vi "RollerTactic.vi"(7 "first call":bool, 8 "error in (no error)":errorcluster, 9 "Robot":refnum<class "Robot.lvclass">, 10 "Game in":refnum<class "Game.lvclass">, 11 "RollerTactic in":refnum<class "RollerTactic.lvclass">) -> (0 "error out":errorcluster, 2 "Robot out":refnum<class "Robot.lvclass">, 3 "RollerTactic out":refnum<class "RollerTactic.lvclass">)   [LabVIEW 2023, in "RollerTactic.lvclass"]
uses:
  RollerTactic.lvclass
  Robot_class/Robot.lvclass
  Game_class/Game.lvclass
  Robot_class/tactics.ctl
  Tactic_class/Tactic.lvclass/Tactic.ctl
  Game_class/Game.lvclass/Game.ctl
  Object_class/Object.lvclass/Object.ctl
  Skillbook_class/Skillbook.lvclass/Skillbook.ctl
  Events_class/Events.lvclass/Events.ctl
  Robot_class/Robot.lvclass/Robot.ctl
  RollerTactic.lvclass/RollerTactic.ctl
  Game_class/Read EventsRef.vi
  Events_class/Read touch.vi
  Skillbook_class/Read KickToSkill.vi
  Game_class/Read BallRef.vi
  Object_class/Read x.vi
  Object_class/Read y.vi
  Tactic_class/Read Skillbook.vi
  Write States.vi
  Robot_class/Write tactic.vi
  Ball_class/Ball.lvclass
  Skillbook_class/Skillbook.lvclass
  Events_class/Events.lvclass
  KickToSkill_class/KickToSkill.lvclass
panel:
  out "x .or. y?":bool
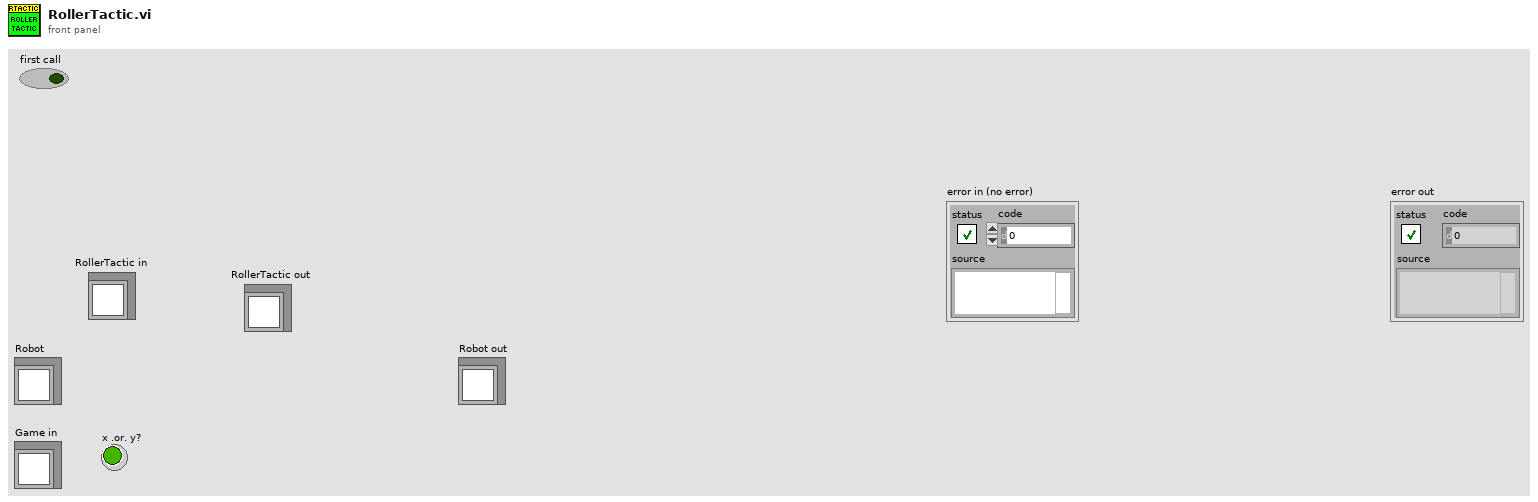
[diagram p1: front panel]
types:
  T1 = typedef "tactics.ctl" = enum16{"ReceivePassInFuturePoint", "Roller", "PrepareRollToPassRollerGoTo", "PrepareRollToPassReceiverGoTo", "WaitRoll", "PositionToRoll", "PenaltyAttacker", "PassObserver", "PenaltyDefense", "TableReceiverTactic", "Test", "DefendGoal", "Marker", "FollowAttacker", "DefendArea", "Shoot", "AttackerAimGoal", "AttackerBallOutOfField", "AttackerBlock", "AttackerStop", "Duelist", "Halt", "ZigZag", "GoTo", "Timeout", "KickToPassReceiver", "PositionToReceivePass", "DefendAreaVSS", "DefendGoalVSS", "KickVSS", "AttackVSS", "DispBallVSS", "PenaltyAttackVSS", "WaitPass"}
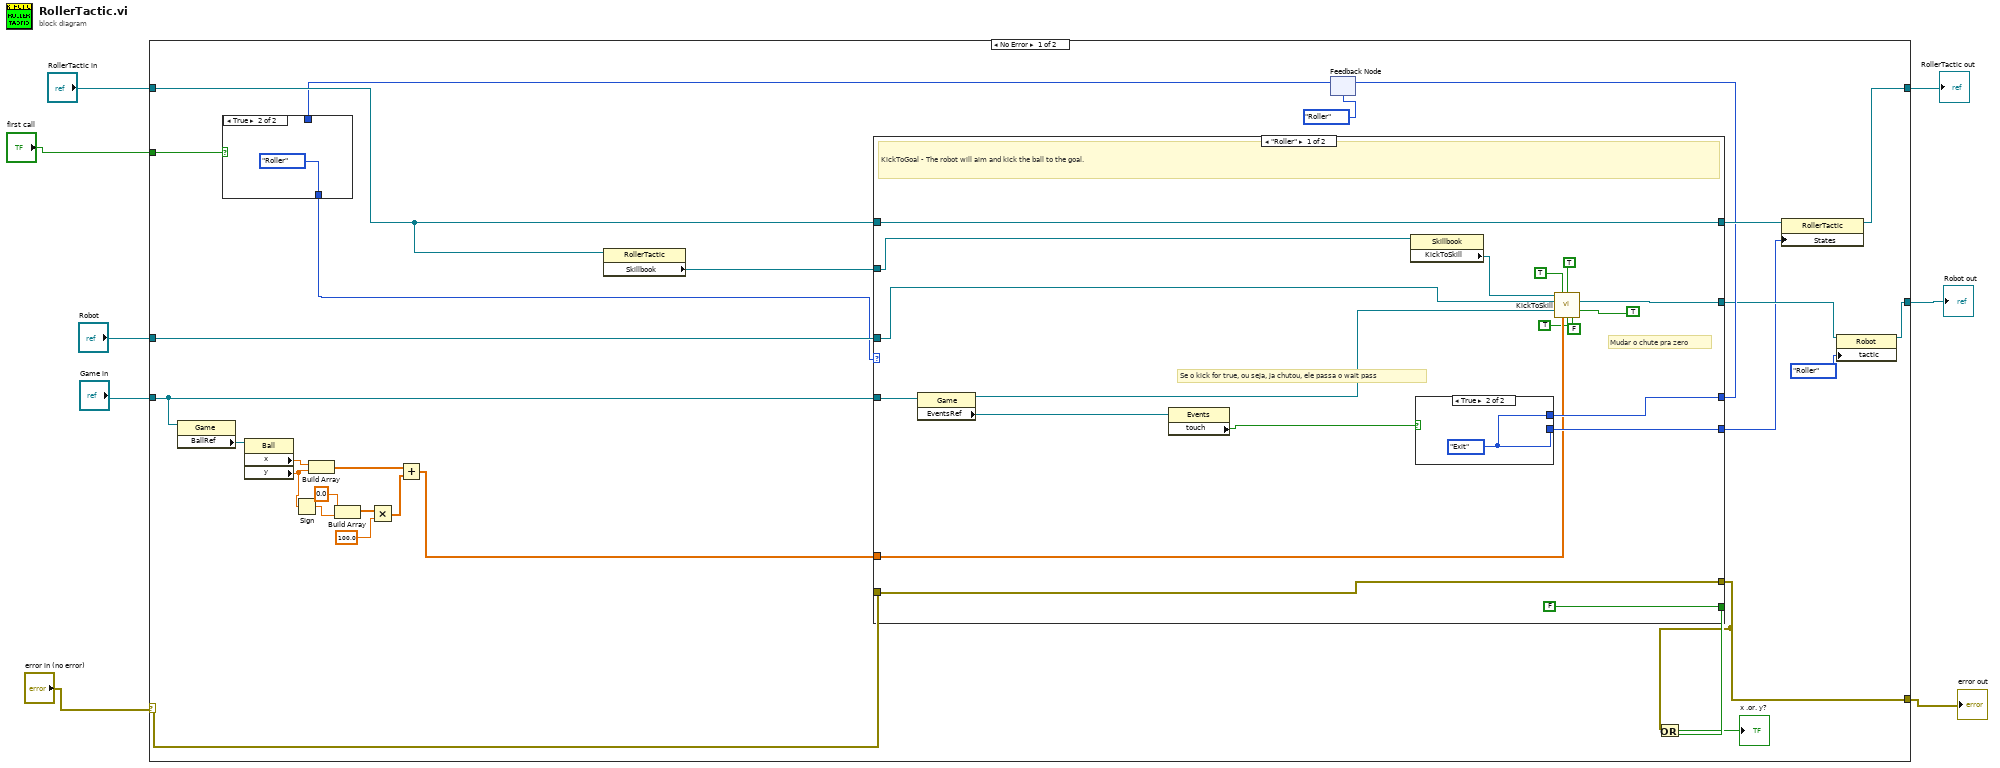
[diagram p0: block diagram]
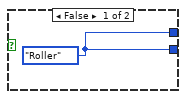
[diagram p3: hidden frame]
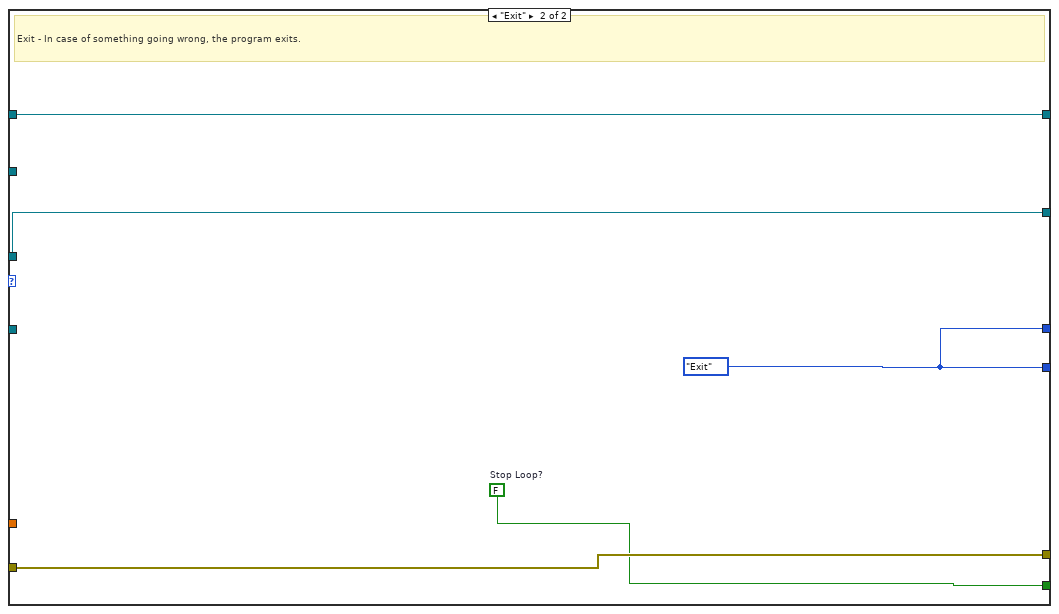
[diagram p4: hidden frame]
diagram:
  n1 = case shown="No Error" "error in (no error)" {
    selector: "error in (no error)" -> [w29 w68]
    tunnel: [w30 w68] -> w4
    tunnel: [w32 w67] -> w1
    tunnel: "RollerTactic in" -> [w33 w67]
    tunnel: "Robot" -> [w31 w66]
    tunnel: "Game in" -> [w28 _]
    tunnel: [w21 w66] -> w6
    tunnel: "first call" -> [w26 _]
    frame No Error {
      n2 = property class="Game"(reference=w28) -> ("BallRef"=w20:refnum<class "Ball.lvclass">)  [unwired: 1 in, 2 out]
      n3 = property class="Ball"(reference=w20) -> ("x"=w19:dbl, "y"=w16:dbl)  [unwired: 1 in, 2 out]
      n4 = Sign(1:w16) -> (0:w15:dbl)
      n5 = Build Array(w19, w16) -> (w18:dbl[])
      n6 = Build Array(0.0 ("element"), w15) -> (w14:dbl[])
      n7 = Multiply(x=w14, y=100.0 ("element")) -> (x*y=w12:dbl[])
      n8 = Add(x=w18, y=w12) -> (x+y=w11:dbl[])
      n9 = property class="RollerTactic"(reference=w33) -> ("Skillbook"=w35:refnum<class "Skillbook.lvclass">)  [unwired: 1 in, 2 out]
      n10 = feedback #1(enum16{"Exit", "Roller"}."Roller" ("States")) -> (w24:enum16{"Exit", "Roller"})
      n11 = case shown="True" w26 {
        tunnel: [w38 enum16{"Exit", "Roller"}."Roller" ("States")] -> w25
        tunnel: w24 -> [w38 _]
        frame False {
        }
        frame True {
        }
      }
      n12 = case shown="\"Roller\"" w25 {
        tunnel: [FALSE ("Stop Loop?") w62] -> w37
        tunnel: w29 -> [w57 w65]
        tunnel: [w57 w65] -> w30
        tunnel: w35 -> [w56 _]
        tunnel: w31 -> [w51 w63]
        tunnel: [w54 w63] -> w22
        tunnel: [w55 w64] -> w34
        tunnel: w33 -> [w55 w64]
        tunnel: w28 -> [w50 _]
        tunnel: [w48 w61] -> w9
        tunnel: [w47 w61] -> w27
        tunnel: w11 -> [w41 _]
        frame "Roller" {
          # "Se o kick for true, ou seja, ja chutou, ele passa o wait pass"
          # "Mudar o chute pra zero"
          # "KickToGoal - The robot will aim and kick the ball to the goal."
          n13 = property class="Game"(reference=w50) -> (reference out=w49:refnum<class "Game.lvclass">, "EventsRef"=w44:refnum<class "Events.lvclass">)  [unwired: 1 in, 1 out]
          n14 = property class="Events"(reference=w44) -> ("touch"=w43:bool)  [unwired: 1 in, 2 out]
          n15 = property class="Skillbook"(reference=w56) -> ("KickToSkill"=w52:refnum<class "KickToSkill.lvclass">)  [unwired: 1 in, 2 out]
          n16 = case shown="True" w43 {
            tunnel: [w59 w60] -> w48
            tunnel: [w59 w60] -> w47
            frame False {
              w59 = enum16{"Exit", "Roller"}."Roller" ("States")
            }
            frame True {
              w60 = enum16{"Exit", "Roller"}."Exit" ("States")
            }
          }
          n17 = call "KickToSkill.vi"("KickToSkill in"=w52, "use criteria?"=TRUE, "chipKick ?"=TRUE, "Robot"=w51, "Game"=w49, "calculate force?"=TRUE, "Target"=w41, "KickForce 0?"=TRUE, "Pass?"=FALSE) -> ("Robot out"=w54:refnum<class "Robot.lvclass">)  [unwired: 4 in, 2 out]
        }
        frame "Exit" {
          w61 = enum16{"Exit", "Roller"}."Exit" ("States")
          w62 = FALSE  # Stop Loop?
          # "Exit - In case of something going wrong, the program exits."
        }
      }
      n18 = feedback-in #1(w27) -> ()
      n19 = Or(x=w30, y=w37) -> (x .or. y?=→"x .or. y?":bool)
      n20 = property class="RollerTactic"(reference=w34, "States"=w9) -> (reference out=w32:refnum<class "RollerTactic.lvclass">)  [unwired: 1 in, 1 out]
      n21 = property class="Robot"(reference=w22, "tactic"=tactics."Roller") -> (reference out=w21:refnum<class "Robot.lvclass">)  [unwired: 1 in, 1 out]
    }
    frame Error {
    }
  }
  "error out" <- w4
  "Robot out" <- w6
  "RollerTactic out" <- w1
